vi "Wait_At_Wire_Err.vi"(8 "InitClock(ms)":u32, 9 "Wait (ms)":u32, 10 "Wait T_Mult(F)":bool, 11 "error in (no error)":errorcluster caption="entrée d'erreur") -> (0 "Clock(ms)":u32, 3 "error out":errorcluster caption="sortie d'erreur", 4 "Delta(ms)":u32)   [LabVIEW 2019]
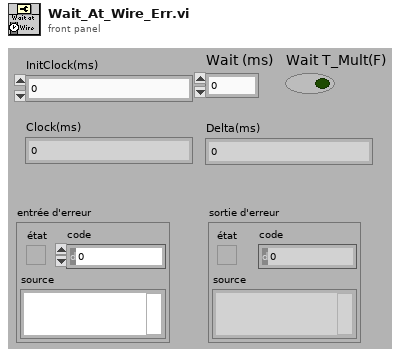
[diagram p1: front panel]
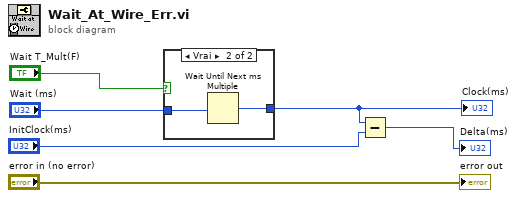
[diagram p0: block diagram]
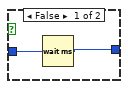
[diagram p2: hidden frame]
diagram:
  n1 = case shown="Vrai" "Wait T_Mult(F)" {
    tunnel: [w8 w10] -> w3
    tunnel: "Wait (ms)" -> [w7 w9]
    frame False {
      n2 = Wait (ms)(milliseconds to wait=w7) -> (millisecond timer value=w8:u32)
    }
    frame True {
      n3 = Wait Until Next ms Multiple(millisecond multiple=w9) -> (millisecond timer value=w10:u32)
    }
  }
  "Clock(ms)" <- w3
  n4 = Subtract(x=w3, y="InitClock(ms)") -> (x-y=→"Delta(ms)":u32)
  "error out" <- "error in (no error)"
